vi "Generate_WayPoints_Hopping_LSV.vi"(11 "Input Cluster":T2={"Scan Rate (um/s)"=15.0, "X Start"=15.0, "X End"=15.0, "Y Start"=15.0, "Y End"=15.0, " Z Start"=15.0, "HoppingDistance"=1.0, "V"=15.0, "Z End"=15.0, "Approach Rate Hopping (um/s)"=15.0, "Retrack Rate (um/s)"=15.0, "V 2"=15.0, "Approach Rate (um/s)"=15.0, "V 3"=15.0, "CV Rate / V/s"=15.0, "V 4"=15.0, "V 1"=15.0, "HoldTime1/s"=15.0, "Hold time 2 / s"=15.0, "Hold time 3/ s"=15.0}) -> (0 "output cluster":T1)   [LabVIEW 2023]
uses:
  TypeDefs/WayPointCluster.ctl
  User_Vi/Settings.vi
panel:
  in  "WayPointCluster":T1
  out "Y  P":dbl
  out "X  P":dbl
  out "HoppingDistanceX":dbl
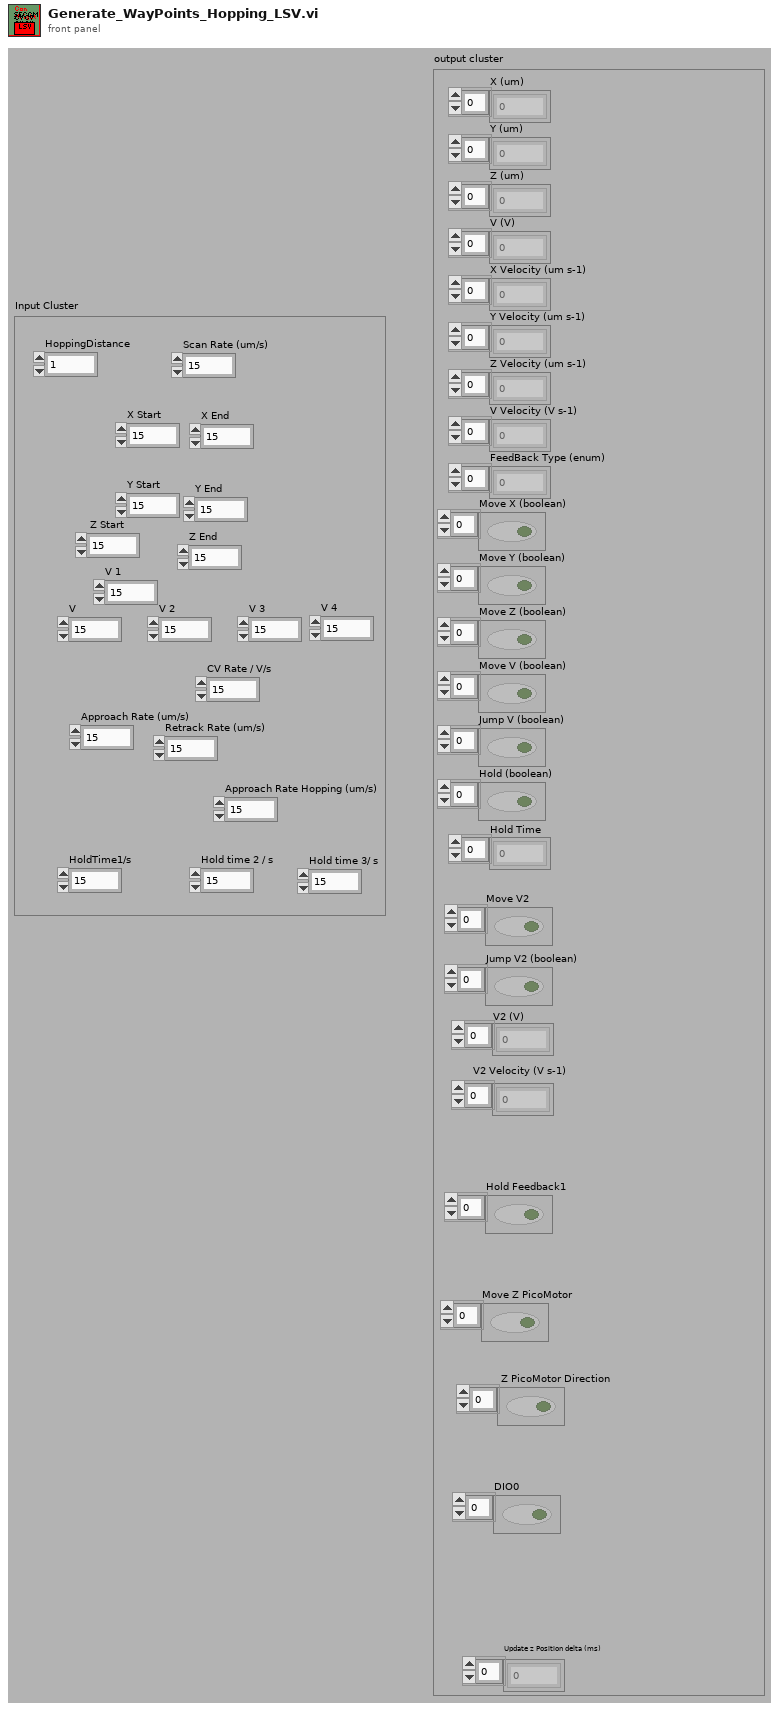
[diagram p1: front panel]
types:
  T1 = typedef "WayPointCluster.ctl" = cluster{"X (um)":dbl[], "Y (um)":dbl[], "Z (um)":dbl[], "V (V)":dbl[], "X Velocity (um s-1)":dbl[], "Y Velocity (um s-1)":dbl[], "Z Velocity (um s-1)":dbl[], "V Velocity (V s-1)":dbl[], "FeedBack Type (enum)":u16[], "Move X (boolean)":bool[], "Move Y (boolean)":bool[], "Move Z (boolean)":bool[], "Move V (boolean)":bool[], "Jump V (boolean)":bool[], "Hold (boolean)":bool[], "Hold Time":u32[], "V2 (V)":dbl[], "Move V2":bool[], "V2 Velocity (V s-1)":dbl[], "Jump V2 (boolean)":bool[], "Update z Position delta (ms)":i16[], "Hold Feedback1":bool[], "Move Z PicoMotor":bool[], " Z PicoMotor Direction":bool[], "DIO0":bool[]}
  T2 = cluster{"Scan Rate (um/s)":dbl, "X Start":dbl, "X End":dbl, "Y Start":dbl, "Y End":dbl, " Z Start":dbl, "HoppingDistance":dbl, "V":dbl, "Z End":dbl, "Approach Rate Hopping (um/s)":dbl, "Retrack Rate (um/s)":dbl, "V 2":dbl, "Approach Rate (um/s)":dbl, "V 3":dbl, "CV Rate / V/s":dbl, "V 4":dbl, "V 1":dbl, "HoldTime1/s":dbl, "Hold time 2 / s":dbl, "Hold time 3/ s":dbl}
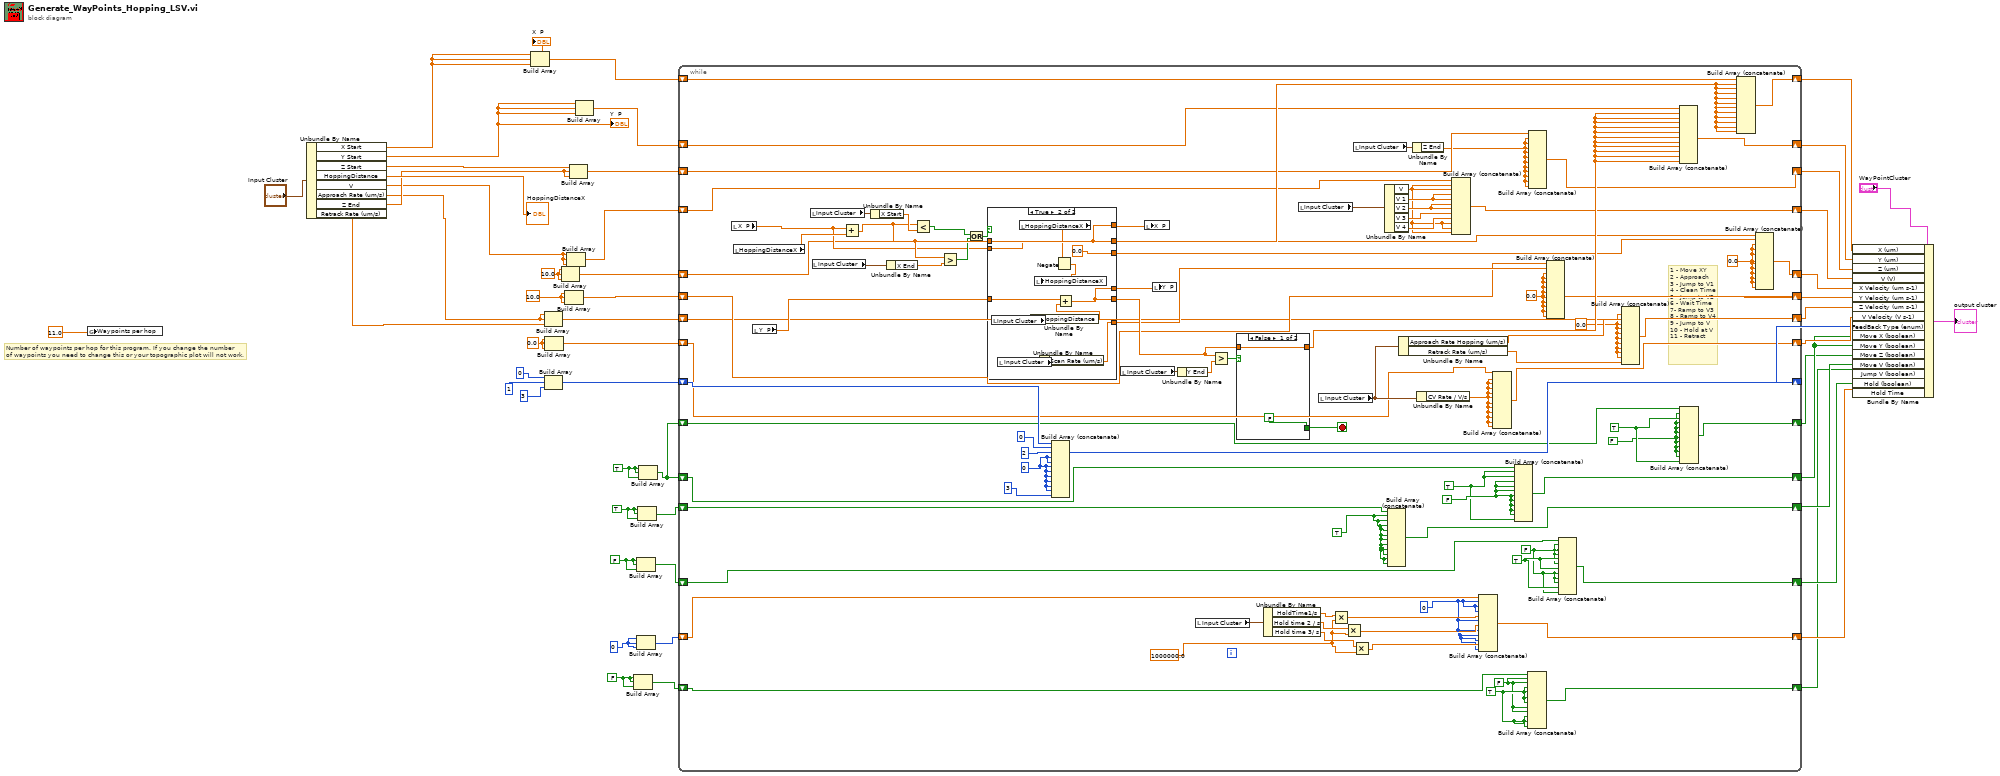
[diagram p0: block diagram]
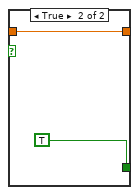
[diagram p2: hidden frame]
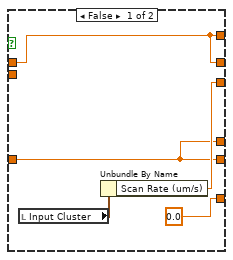
[diagram p3: hidden frame]
diagram:
  w13 = FALSE
  w17 = FALSE
  w16 = u32 0 ("element")
  w15 = TRUE
  w11 = TRUE
  w7 = 10.0 ("element")
  w8 = 10.0 ("element")
  w10 = 0.0 ("element")
  # "Number of waypoints per hop for this program. If you change the number\nof waypoints you need to change this or your topographic plot will not work."
  n1 = global write "Settings.vi" "Waypoints per hop"(11.0) -> ()
  n2 = Unbundle By Name("Input Cluster") -> ("X Start"=w31:dbl, "Y Start"=w30:dbl, "Z Start"=w32:dbl, "HoppingDistance"=→"HoppingDistanceX":dbl, "V"=w28:dbl, "Approach Rate (um/s)"=w9:dbl, "Z End"=w29:dbl, "Retrack Rate (um/s)"=w27:dbl)
  "X  P" <- w31
  "Y  P" <- w30
  n3 = Build Array(w31, w31, w31) -> (w50:dbl[])
  n4 = Build Array(w9, w9, w27) -> (w39:dbl[])
  n5 = Build Array(u16 0 ("element"), u16 1 ("element"), u16 3 ("element")) -> (w35:u16[])
  n6 = Build Array(w10, w10, w10) -> (w37:dbl[])
  n7 = Build Array(w7, w7, w7) -> (w42:dbl[])
  n8 = Build Array(w8, w8, w8) -> (w41:dbl[])
  n9 = Build Array(w28, w28, w28) -> (w44:dbl[])
  n10 = Build Array(w32, w29, w29) -> (w46:dbl[])
  n11 = Build Array(w30, w30, w30) -> (w48:dbl[])
  n12 = Build Array(w17, w17, w17) -> (w20:bool[])
  n13 = Build Array(w13, w13, w13) -> (w12:bool[])
  n14 = Build Array(w16, w16, w16) -> (w24:u32[])
  n15 = Build Array(w15, w15, w15) -> (w19:bool[])
  n16 = Build Array(w11, w11, w11) -> (w3:bool[])
  n17 = while {
    shift-right: [w113] -> w49
    shift-left: w50 -> [w114]
    shift-right: [w110] -> w47
    shift-left: w48 -> [w111]
    shift-right: [w107] -> w45
    shift-left: w46 -> [w108]
    shift-right: [w97] -> w43
    shift-left: w44 -> [w98]
    shift-right: [w91] -> w25
    shift-left: w42 -> [w105]
    shift-right: [w100] -> w40
    shift-left: w41 -> [w101]
    shift-right: [w90] -> w38
    shift-left: w39 -> [w57]
    shift-right: [w60] -> w36
    shift-left: w37 -> [w86]
    shift-right: [w137] -> w34
    shift-left: w35 -> [w138]
    shift-right: [w83] -> w23
    shift-left: w3 -> [w84]
    shift-right: [w76] -> w22
    shift-left: w12 -> [w77]
    shift-right: [w72] -> w21
    shift-left: w24 -> [w73]
    shift-right: [w62] -> w4
    shift-left: w20 -> [w63]
    shift-right: [w79] -> w14
    shift-left: w19 -> [w80]
    shift-right: [w55] -> w2
    shift-left: w3 -> [w54]
    stop <- w125 stop-if-true
    w53 = FALSE
    w56 = TRUE
    w58 = 1000000.0 ("y")
    w61 = TRUE
    w103 = 0.0 ("element")
    w78 = TRUE
    w59 = FALSE
    w64 = u32 0 ("element")
    w75 = TRUE
    w74 = FALSE
    w82 = FALSE
    w81 = TRUE
    w116 = u16 0 ("element")
    w99 = 0.0 ("element")
    w88 = 0.0 ("element")
    # "1 - Move XY\n2 - Approach\n3 - Jump to V1\n4 - Clean Time\n5 - Jump to V2\n6 - Wait Time\n7- Ramp to V3\n8 - Ramp to V4\n9 - Jump to V\n10 - Hold at V\n11 - Retract"
    n18 = local read "X  P"() -> (w124:dbl)
    n19 = local read "HoppingDistanceX"() -> (w139:dbl)
    n20 = local read "Y  P"() -> (w123:dbl)
    n21 = local read "Input Cluster"() -> (w141:T2)
    n22 = local read "Input Cluster"() -> (w140:T2)
    n23 = Add(x=w124, y=w139) -> (x+y=w131:dbl)
    n24 = Unbundle By Name(w141) -> ("X Start"=w134:dbl)
    n25 = Unbundle By Name(w140) -> ("X End"=w132:dbl)
    n26 = Less?(x=w131, y=w134) -> (x < y?=w133:bool)
    n27 = Greater?(x=w131, y=w132) -> (0:w130:bool)
    n28 = Or(x=w133, y=w130) -> (x .or. y?=w129:bool)
    n29 = case shown="True" w129 {
      tunnel: w131 -> [w146 _]
      tunnel: [w146 w152] -> w112
      tunnel: w124 -> [_ w152]
      tunnel: w123 -> [w147 w153]
      tunnel: [w147 w151] -> w122
      tunnel: [w149 0.0] -> w104
      tunnel: [0.0 w154] -> w102
      tunnel: [w147 w151] -> w121
      tunnel: [w146 w152] -> w120
      frame False {
        n30 = local read "Input Cluster"() -> (w150:T2)
        n31 = Unbundle By Name(w150) -> ("Scan Rate (um/s)"=w149:dbl)
      }
      frame True {
        n32 = local read "Input Cluster"() -> (w158:T2)
        n33 = local read "Input Cluster"() -> (w156:T2)
        n34 = local read "HoppingDistanceX"() -> (w160:dbl)
        n35 = Unbundle By Name(w158) -> ("HoppingDistance"=w157:dbl)
        n36 = Unbundle By Name(w156) -> ("Scan Rate (um/s)"=w154:dbl)
        n37 = Negate(x=w160) -> (-x=w159:dbl)
        n38 = local write "HoppingDistanceX"(w159) -> ()
        n39 = Add(x=w153, y=w157) -> (x+y=w151:dbl)
      }
    }
    n40 = Build Array (concatenate)(w138, u16 0 ("element"), u16 2 ("element"), w116, w116, w116, w116, w116, w116, w116, w116, u16 3 ("element")) -> (w137:u16[])
    n41 = local read "Input Cluster"() -> (w128:T2)
    n42 = local write "X  P"(w120) -> ()
    n43 = local write "Y  P"(w121) -> ()
    n44 = Unbundle By Name(w128) -> ("Y End"=w127:dbl)
    n45 = local read "Input Cluster"() -> (w71:T2)
    n46 = Greater?(x=w122, y=w127) -> (0:w126:bool)
    n47 = case shown="False" w126 {
      tunnel: w122 -> [w143 w145]
      tunnel: [w143 w145] -> w109
      tunnel: [FALSE TRUE] -> w125
      frame False {
      }
      frame True {
      }
    }
    n48 = Unbundle By Name(w71) -> ("HoldTime1/s"=w70:dbl, "Hold time 2 / s"=w69:dbl, "Hold time 3/ s"=w68:dbl)
    n49 = local read "Input Cluster"() -> (w135:T2)
    n50 = local read "Input Cluster"() -> (w117:T2)
    n51 = Multiply(x=w70, y=w58) -> (x*y=w67:dbl)
    n52 = Multiply(x=w69, y=w58) -> (x*y=w66:dbl)
    n53 = Multiply(x=w68, y=w58) -> (x*y=w65:dbl)
    n54 = local read "Input Cluster"() -> (w136:T2)
    n55 = Unbundle By Name(w135) -> ("V"=w92:dbl, "V 1"=w96:dbl, "V 2"=w95:dbl, "V 3"=w94:dbl, "V 4"=w93:dbl)
    n56 = Build Array (concatenate)(w80, w78, w78, w78, w78, w78, w78, w78, w78, w78, w78, w78) -> (w79:bool[])
    n57 = Unbundle By Name(w117) -> ("Approach Rate Hopping (um/s)"=w89:dbl, "Retrack Rate (um/s)"=w87:dbl)
    n58 = Unbundle By Name(w136) -> ("Z End"=w106:dbl)
    n59 = Unbundle By Name(w117) -> ("CV Rate / V/s"=w85:dbl)
    n60 = Build Array (concatenate)(w98, w92, w92, w96, w96, w95, w95, w94, w93, w92, w92, w92) -> (w97:dbl[])
    n61 = Build Array (concatenate)(w73, w64, w64, w64, w67, w64, w66, w64, w64, w64, w65, w64) -> (w72:dbl[])
    n62 = Build Array (concatenate)(w86, w85, w85, w85, w85, w85, w85, w85, w85, w85, w85, w85) -> (w60:dbl[])
    n63 = Build Array (concatenate)(w84, w81, w81, w82, w82, w82, w82, w82, w82, w82, w82, w81) -> (w83:bool[])
    n64 = Build Array (concatenate)(w63, w59, w59, w61, w61, w61, w61, w59, w59, w61, w61, w61) -> (w62:bool[])
    n65 = Build Array (concatenate)(w108, w106, w106, w106, w106, w106, w106, w106, w106, w106, w106, w106) -> (w107:dbl[])
    n66 = Build Array (concatenate)(w101, w102, w99, w99, w99, w99, w99, w99, w99, w99, w99, w99) -> (w100:dbl[])
    n67 = Build Array (concatenate)(w77, w74, w74, w74, w75, w74, w75, w74, w74, w74, w75, w74) -> (w76:bool[])
    n68 = Build Array (concatenate)(w57, w88, w89, w88, w88, w88, w88, w88, w88, w88, w88, w87) -> (w90:dbl[])
    n69 = Build Array (concatenate)(w111, w109, w109, w109, w109, w109, w109, w109, w109, w109, w109, w109) -> (w110:dbl[])
    n70 = Build Array (concatenate)(w54, w53, w56, w53, w53, w53, w53, w53, w53, w53, w53, w56) -> (w55:bool[])
    n71 = Build Array (concatenate)(w114, w112, w112, w112, w112, w112, w112, w112, w112, w112, w112, w112) -> (w113:dbl[])
    n72 = Build Array (concatenate)(w105, w104, w103, w103, w103, w103, w103, w103, w103, w103, w103, w103) -> (w91:dbl[])
  }
  n73 = Bundle By Name(cluster="WayPointCluster", "X (um)"=w49, "Y (um)"=w47, "Z (um)"=w45, "V (V)"=w43, "X Velocity (um s-1)"=w25, "Y Velocity (um s-1)"=w40, "Z Velocity (um s-1)"=w38, "V Velocity (V s-1)"=w36, "FeedBack Type (enum)"=w34, "Move X (boolean)"=w23, "Move Y (boolean)"=w23, "Move Z (boolean)"=w2, "Move V (boolean)"=w14, "Jump V (boolean)"=w4, "Hold (boolean)"=w22, "Hold Time"=w21) -> (→"output cluster":T1)
